vi "TCP-pack.vi"(2 "Data to send":string) -> (6 "Data toTCP":string)   [LabVIEW 2020, in "Sgraph_lib_V1.lvlib"]
doc: "TCP compose string for sending\nMake datagram from string header and size"
uses:
  Builds/Sgraph_lib_V1.lvlib
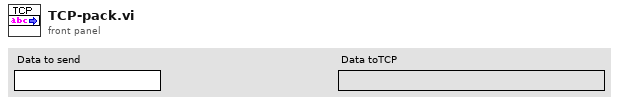
[diagram p1: front panel]
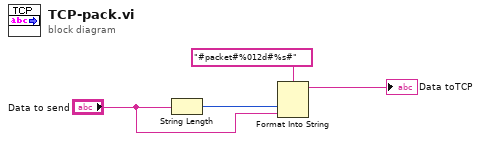
[diagram p0: block diagram]
diagram:
  n1 = String Length(string="Data to send") -> (length=w3:i32)
  n2 = Format Into String(format string="#packet#%012d#%s#", w3, "Data to send") -> (resulting string=→"Data toTCP":string)  [unwired: 2 in, 1 out]
